vi "Get Class Instance.vi"() -> (3 "Classes":string[](array[string]))   [LabVIEW 2020]
uses:
  Class/OsciloscopeClass/OsciloscopeClass.lvclass
  Class/Tektroniks/Tektronicks.lvclass
  C:/Users/HP/Desktop/Osciloscope/Class/OsciloscopeClass/OsciloscopeClass.lvclass
  Class/EDU-X 1002A/EDU-X 1002A.lvclass
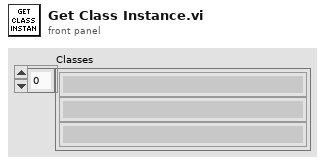
[diagram p1: front panel]
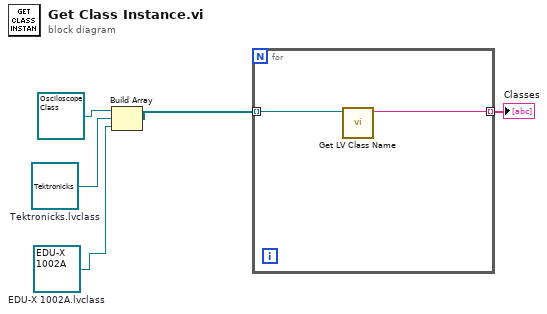
[diagram p0: block diagram]
diagram:
  w1 = refnum<class "EDU-X 1002A.lvclass"> refnum  # EDU-X 1002A.lvclass
  w2 = refnum<class "Tektronicks.lvclass"> refnum  # Tektronicks.lvclass
  n1 = Build Array(refnum<class "OsciloscopeClass.lvclass"> refnum ("OsciloscopeClass.lvclass"), w2, w1) -> (w4:refnum<class "OsciloscopeClass.lvclass">[])
  n2 = for {
    tunnel: w4 -> [w6] mode=indexing
    tunnel: [w7] -> w5 mode=indexing
    n3 = call <vilib>:"Get LV Class Name.vi"("object"=w6) -> ("class name"=w7:string)  [unwired: 9 in, 1 out]
  }
  "Classes" <- w5
